vi "Add User.vi"(10 "User Type":string, 11 "Path":path=path "E:/labview code/project user login/test1.txt") -> (3 "output data":string[][](array[string]))   [LabVIEW 2015]
panel:
  in  "SELECT USER TYPE":u16(ring) items=["Supervisor", "Operator"]
  in  "Add Button":bool
  in  "Password":string
  in  "User Name":string
  # "* Mandatory Field (Minimum length 4)"
  # "* Mandatory Field (Minimum length 4)"
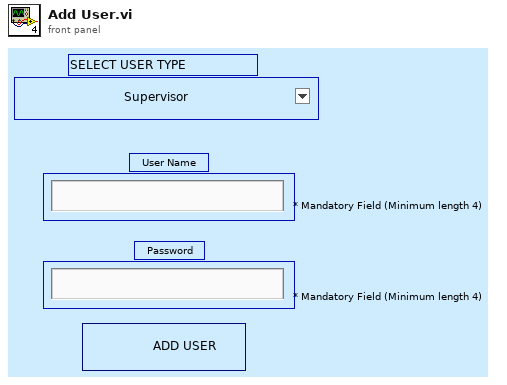
[diagram p1: front panel]
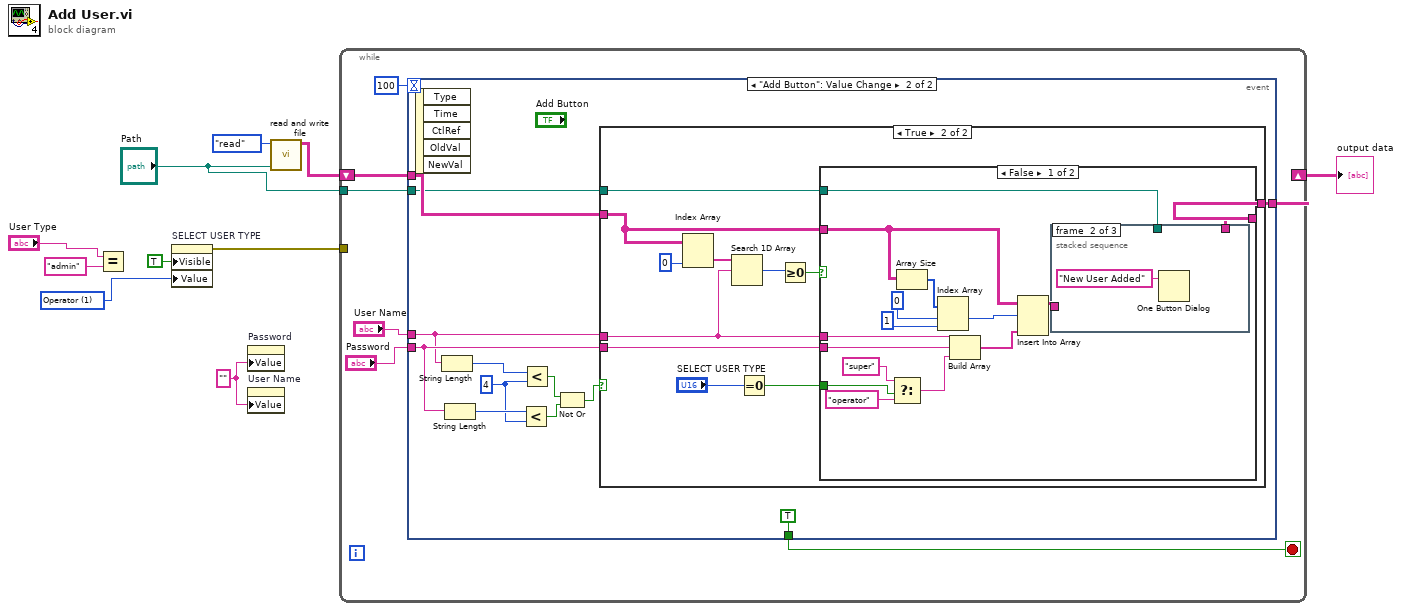
[diagram p0: block diagram]
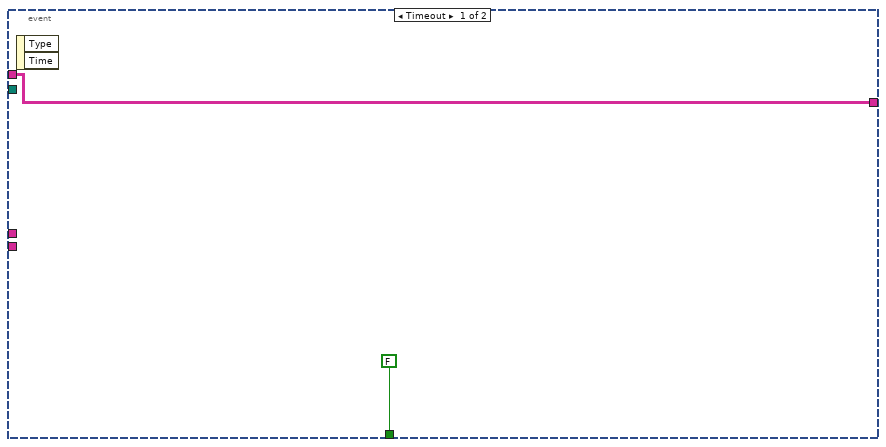
[diagram p2: hidden frame]
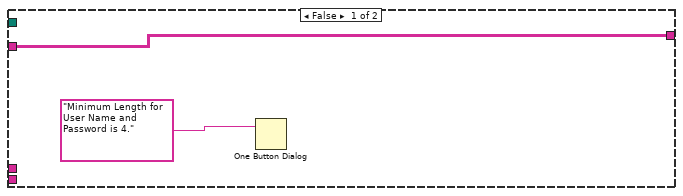
[diagram p3: hidden frame]
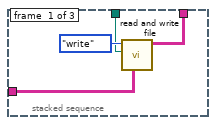
[diagram p4: hidden frame]
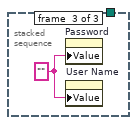
[diagram p5: hidden frame]
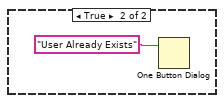
[diagram p6: hidden frame]
diagram:
  w3 = u16 1 items=["Supervisor", "Operator"] ("SELECT USER TYPE")
  w7 = "" ("User Name")
  n1 = Equal?(x="User Type", y="admin") -> ()  [unwired: 1 out]
  n2 = property on="SELECT USER TYPE" class="Ring (strict)"("Visible"=TRUE, "Value"=w3) -> (error out=w2:errorcluster)  [unwired: 2 in, 1 out]
  n3 = property on="Password" class="Str"("Value"=w7) -> ()  [unwired: 2 in, 2 out]
  n4 = property on="User Name" class="Str"("Value"=w7) -> ()  [unwired: 2 in, 2 out]
  n5 = call "read and write file.vi"("Path"="Path", "Enum"=enum16{"write", "read"}."read") -> ("output data"=w9:string[][])  [unwired: 9 in]
  n6 = while {
    shift-right: [w15] -> w8
    shift-left: w9 -> [w16]
    tunnel: "Path" -> [w11]
    tunnel: w2 -> [_]
    stop <- w17 stop-if-true
    n7 = event shown="[1] \"Add Button\": Value Change" {
      selector: _ -> [_ _]
      dyn-events: _ -> [_ _]
      timeout: 100 -> [_ _]
      tunnel: [FALSE ("Exit 2") TRUE ("Exit 2")] -> w17
      tunnel: w16 -> [w19 w30]
      tunnel: [w19 w31] -> w15
      tunnel: "User Name" -> [_ w25]
      tunnel: "Password" -> [_ w29]
      tunnel: w11 -> [_ w26]
      event Timeout {
        n8 = event-data() -> ()  [unwired: 1 in, 2 out]
      }
      event "Add Button": Value Change {
        w22 = 4 ("y")
        n9 = event-data() -> ()  [unwired: 1 in, 5 out]
        n10 = String Length(string=w25) -> (length=w24:i32)
        n11 = String Length(string=w29) -> (length=w23:i32)
        n12 = Less?(x=w23, y=w22) -> (x < y?=w28:bool)
        n13 = Less?(x=w24, y=w22) -> (x < y?=w21:bool)
        n14 = Not Or(1:w28, 2:w21) -> (0:w27:bool)
        n15 = case shown="True" w27 {
          tunnel: [w33 w44] -> w31
          tunnel: w29 -> [_ w43]
          tunnel: w30 -> [w33 w39]
          tunnel: w25 -> [_ w37]
          tunnel: w26 -> [_ w36]
          frame False {
            n16 = One Button Dialog(message="Minimum Length for User Name and Password is 4." ("f")) -> ()  [unwired: 1 in, 1 out]
          }
          frame True {
            n17 = Index Array(array=w39, index (col)=0 ("index (row)")) -> (element=w41:string[])  [unwired: 1 in]
            n18 = Search 1D Array(1D array=w41, element=w37) -> (index of element=w40:i32)  [unwired: 1 in]
            n19 = Equal To 0?(x="SELECT USER TYPE") -> (x = 0?=w34:bool)
            n20 = Greater Or Equal To 0?(x=w40) -> (x >= 0?=w38:bool)
            n21 = case shown="False" w38 {
              tunnel: [w53 _] -> w44
              tunnel: w37 -> [w52 _]
              tunnel: w43 -> [w51 _]
              tunnel: w39 -> [w50 _]
              tunnel: w36 -> [w49 _]
              tunnel: w34 -> [w45 _]
              frame False {
                n22 = Select(t="super" ("element"), s=w45, f="operator" ("element")) -> (s? t:f=w46:string)
                n23 = Array Size(array=w50) -> (size(s)=w59:i32[])
                n24 = Index Array(array=w59, index #1=0 ("index"), index #2=1 ("index")) -> (element #1=w55:i32)  [unwired: 1 out]
                n25 = Build Array(w52, w51, w46) -> (w56:string[])
                n26 = Insert Into Array(array=w50, index (row)=w55, new element=w56) -> (w54:string[][])  [unwired: 1 in]
                n27 = stacked-sequence {
                  tunnel: w54 -> [w63 _ _]
                  tunnel: [w61 _ _] -> w53
                  tunnel: w49 -> [w60 _ _]
                  frame #0 {
                    n28 = call "read and write file.vi"("data to write"=w63, "Path"=w60, "Enum"=enum16{"write", "read"}."write") -> ("output data"=w61:string[][])  [unwired: 8 in]
                  }
                  frame #1 {
                    n29 = One Button Dialog(message="New User Added") -> ()  [unwired: 1 in, 1 out]
                  }
                  frame #2 {
                    w65 = "" ("User Name")
                    n30 = property on="Password" class="Str"("Value"=w65) -> ()  [unwired: 2 in, 2 out]
                    n31 = property on="User Name" class="Str"("Value"=w65) -> ()  [unwired: 2 in, 2 out]
                  }
                }
              }
              frame True {
                n32 = One Button Dialog(message="User Already Exists") -> ()  [unwired: 1 in, 1 out]
              }
            }
          }
        }
      }
    }
  }
  "output data" <- w8
